vi "measure DAQ voltage output speed.vi"() -> ()   [LabVIEW 2021]
panel:
  out "x-y":dbl
  out "relative seconds":dbl format="%_19f"
  out "start time s":dbl format="%_19f"
  in  "Physical Channel(s)":tag="Dev3/ao0"
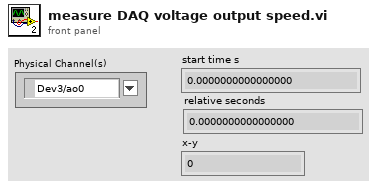
[diagram p1: front panel]
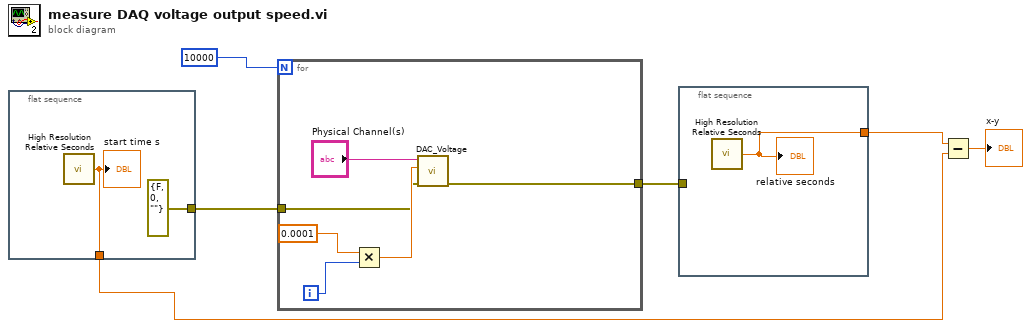
[diagram p0: block diagram]
diagram:
  n1 = flat-sequence {
    tunnel: [errorcluster {"status"=FALSE, "code"=0, "source"=""} ("error in")] -> w5
    tunnel: [w7] -> w2
    frame #0 {
      n2 = call <vilib>:"High Resolution Relative Seconds.vi"() -> ("relative seconds"=w7:dbl)
      "start time s" <- w7
    }
  }
  n3 = for {
    N: 10000 -> [_]
    tunnel: w5 -> [w10]
    tunnel: [w9] -> w4
    i -> [w14]
    n4 = Multiply(x=0.0001, y=w14) -> (x*y=w12:dbl)
    n5 = call "DAC_Voltage.vi"("error in"=w10, "Voltage"=w12, "Physical Channel(s)"="Physical Channel(s)") -> ("error out"=w9:errorcluster)  [unwired: 8 in]
  }
  n6 = flat-sequence {
    tunnel: w4 -> [_]
    tunnel: [w15] -> w3
    frame #0 {
      n7 = call <vilib>:"High Resolution Relative Seconds.vi"() -> ("relative seconds"=w15:dbl)
      "relative seconds" <- w15
    }
  }
  n8 = Subtract(x=w3, y=w2) -> (x-y=→"x-y":dbl)
